vi "Actor Core.vi"(8 "error in":errorcluster, 11 "Controller in":refnum<class "Controller.lvclass">) -> (0 "error out":errorcluster, 3 "Actor out":refnum<class "Actor.lvclass">)   [LabVIEW 2016, in "Controller.lvlib" / "Controller.lvclass"]
doc: "(<B>Filename</B>: Actor Framework.lvlib:Actor.lvclass:Actor Core.vi)\n\nReceives messages to the actor, reacts to them, and initiates any error handling that may shut the actor down.\n\nDescendant classes may override this VI to append parallel tasks for the actor to complete while it handles messages. Overrides use the Call Parent Method node."
uses:
  Controller.lvclass
  C:/Program Files (x86)/National Instruments/LabVIEW 2016/vi.lib/ActorFramework/Actor/Actor.lvclass
  <vilib>/ActorFramework/Actor/Actor.lvclass
  Controls/Controller States.ctl
  Controls/Controller Data.ctl
  <vilib>/ActorFramework/Message Enqueuer/Message Enqueuer.lvclass
  UI/UI/Controls/Start Acquisition.ctl
  <vilib>/userdefined/High Color/IMAQdx.ctl
  Controller.lvclass/Controller.ctl
  Controls/List of Nested Actors.ctl
  UI/UI/UI.lvclass
  <vilib>/ActorFramework/Actor/Actor.lvclass/Actor.ctl
  <vilib>/ActorFramework/Message Enqueuer/Message Enqueuer.lvclass/Message Enqueuer.ctl
  Image Acquisition/Image Acquisition/Image Acquisition.lvclass
  Image Acquisition/Image Acquisition Messages/Start Acq Msg/Start Acq Msg.lvclass/Start Acq Msg.ctl
  Controller Messages/UpdateAcquisitionEnqueuer Msg/UpdateAcquisitionEnqueuer Msg.lvclass/UpdateAcquisitionEnqueuer Msg.ctl
  Tests/Tests/Child Classes/Threshold/Threshold.lvclass
  Tests/Tests/Child Classes/Grayscale/Grayscale.lvclass
  Tests/Tests/Child Classes/Histogram/Histogram.lvclass
  <vilib>/ActorFramework/Report Error Msg/Report Error Msg.lvclass/Report Error Msg.ctl
  <vilib>/ActorFramework/Message Enqueuer/Init from Existing Queue.vi
  <vilib>/ActorFramework/Message Enqueuer/Enqueue.vi
  Image Acquisition/Image Acquisition Messages/Start Acq Msg/Start Acq Msg.lvclass
  C:/Program Files (x86)/National Instruments/LabVIEW 2016/vi.lib/ActorFramework/Message/Message.lvclass
  Controller Messages/UpdateAcquisitionEnqueuer Msg/UpdateAcquisitionEnqueuer Msg.lvclass
  Image Acquisition/Image Acquisition Messages/Stop Acq Msg/Stop Acq Msg.lvclass
  <vilib>/ActorFramework/Report Error Msg/Report Error Msg.lvclass
  <vilib>/ActorFramework/Stop Msg/Stop Msg.lvclass
  <vilib>/ActorFramework/Message Priority Queue/Priority Enqueue.vi
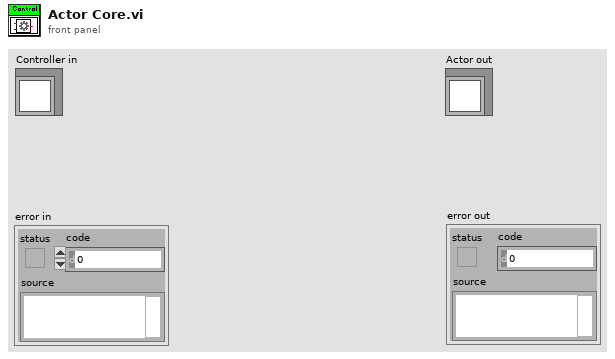
[diagram p1: front panel]
types:
  T1 = typedef "Controller Data.ctl" = cluster{"Controller in":refnum<class "Controller.lvclass">, "Self Enqueuer":refnum<class "Message Enqueuer.lvclass">, "ImgAcq Enqueuer":refnum<class "Message Enqueuer.lvclass">, "UI Enqueuer":refnum<class "Message Enqueuer.lvclass">, "Event Reg Refnum":refnum<event-registration>, "Start Acquisition":T2, "Grayscale Enqueuers":refnum<class "Message Enqueuer.lvclass">[], "HIstogram Enqueuers":refnum<class "Message Enqueuer.lvclass">[], "Threshold Enqueuers":refnum<class "Message Enqueuer.lvclass">[]}
  T2 = typedef "Start Acquisition.ctl" = cluster{"Image Indicator Reference":refnum<vi>, "Start":bool, "Camera":T3}
  T3 = typedef "IMAQdx.ctl" = refnum<k21>
  T4 = typedef "Controller States.ctl" = enum16{"Poll", "Initialize", "Launch-ImgAcqActor", "Stop-ImgAcqActor", "Launch-Threshold", "Launch-Grayscale", "Launch-Histogram", "Stop-Threshold", "Stop-Histogram", "Stop-Grayscale", "Error", "Exit"}
  T5 = typedef "List of Nested Actors.ctl" = enum16{"Threshold", "Grayscale", "Histogram", "UI", "Acquisition"}
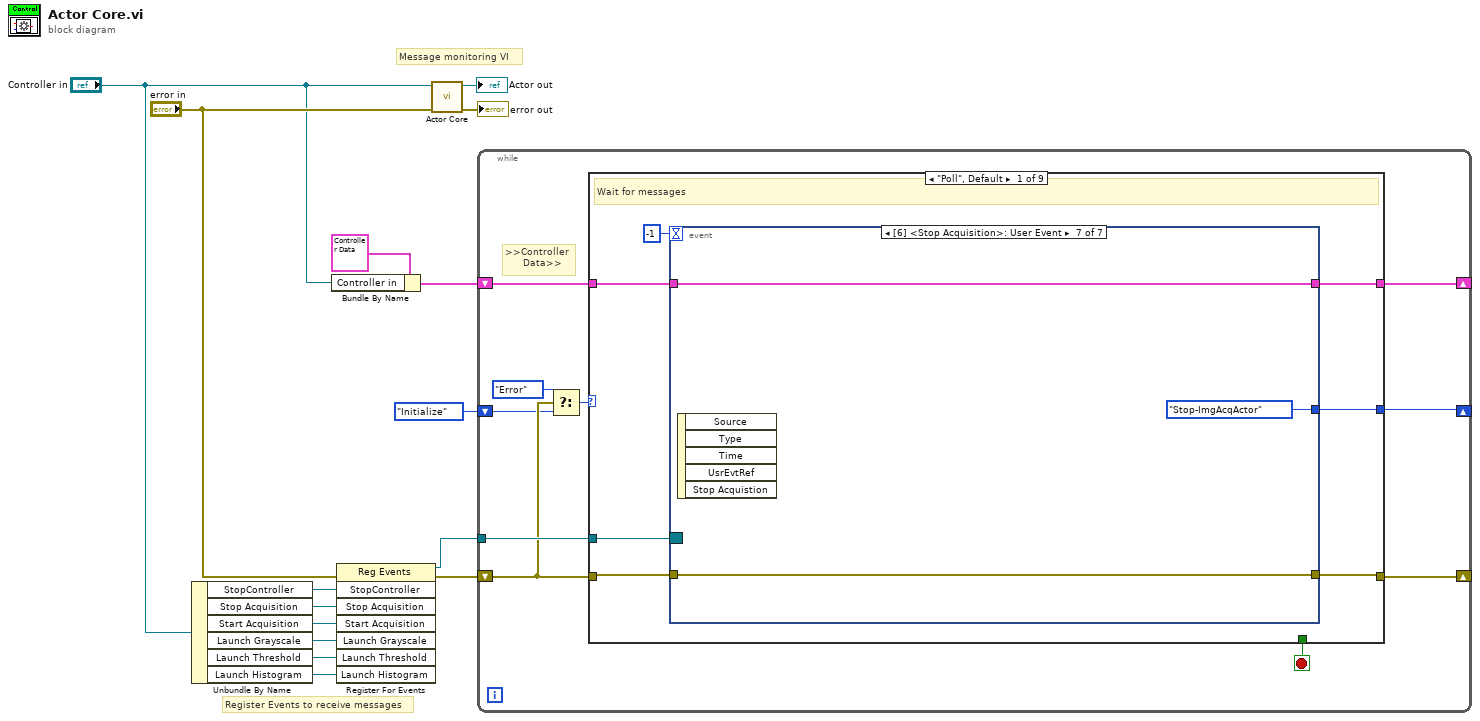
[diagram p0: block diagram]
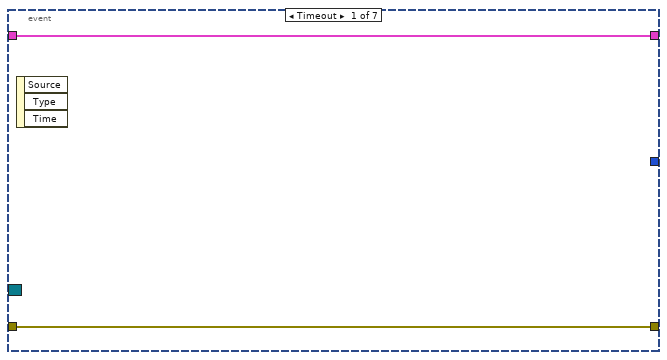
[diagram p2: hidden frame]
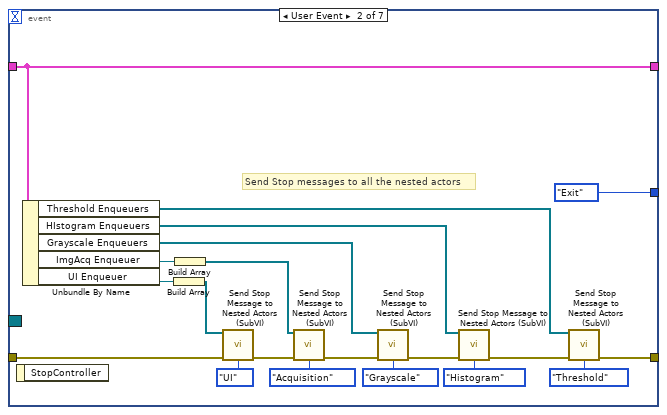
[diagram p3: hidden frame]
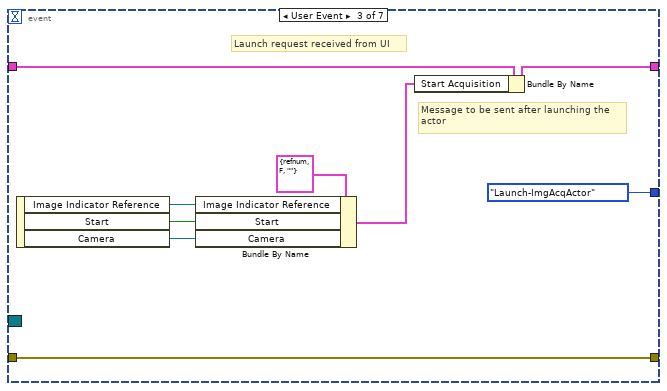
[diagram p4: hidden frame]
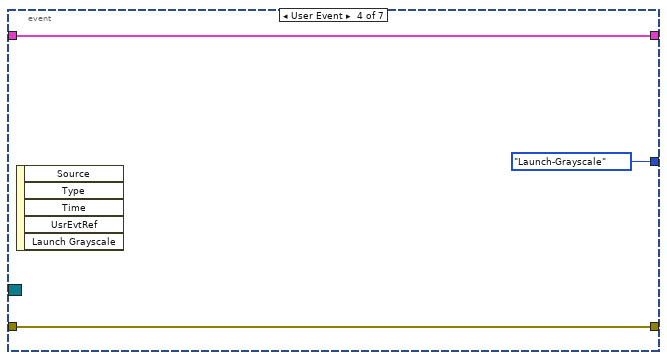
[diagram p5: hidden frame]
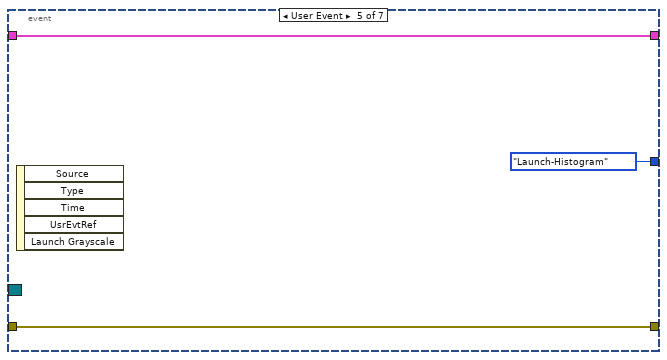
[diagram p6: hidden frame]
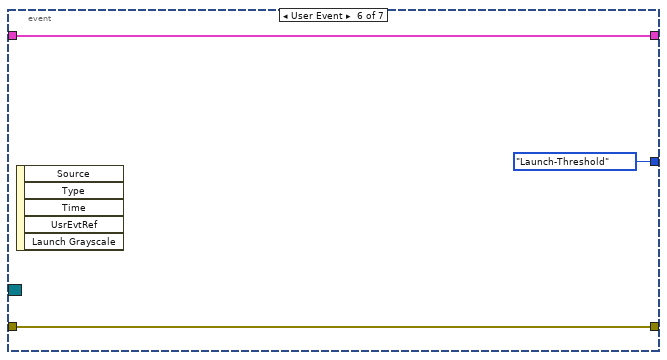
[diagram p7: hidden frame]
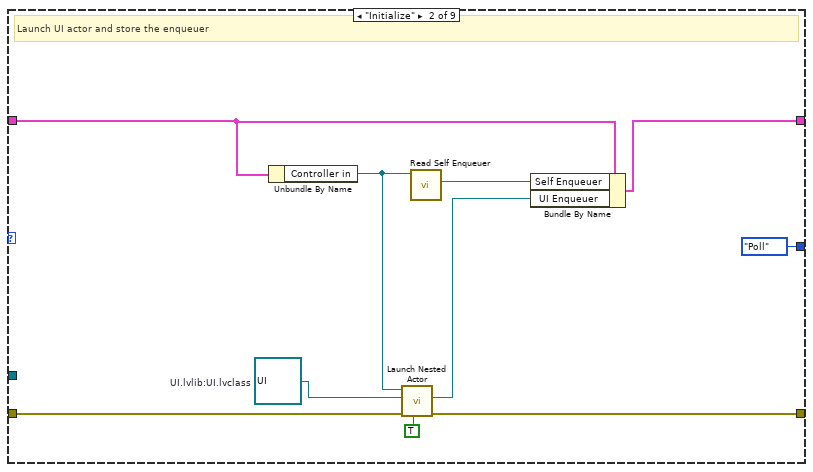
[diagram p8: hidden frame]
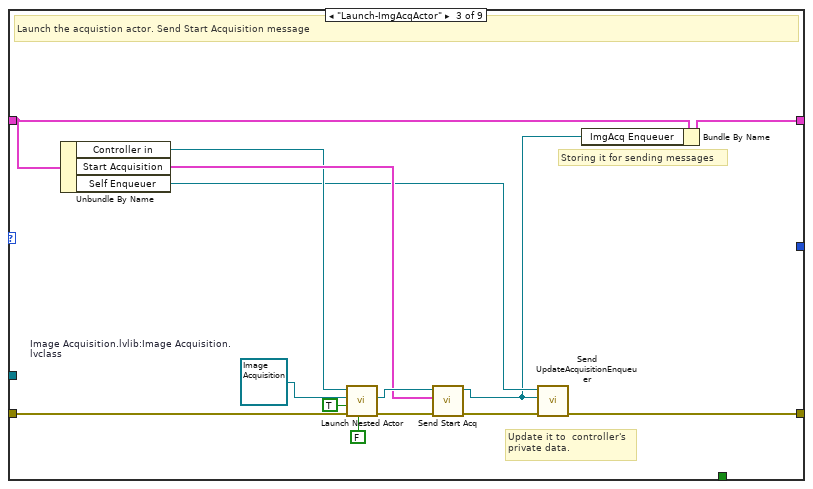
[diagram p9: hidden frame]
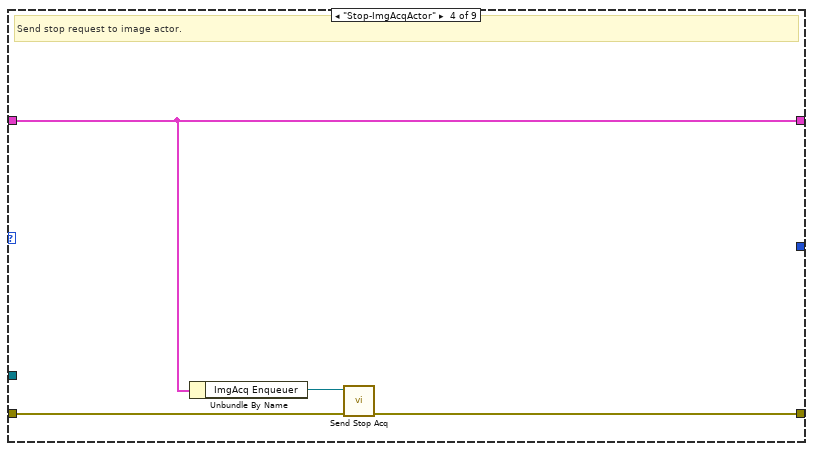
[diagram p10: hidden frame]
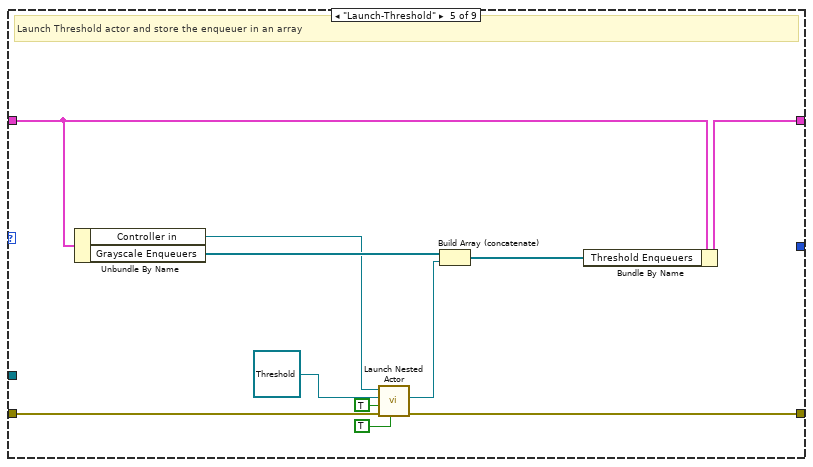
[diagram p11: hidden frame]
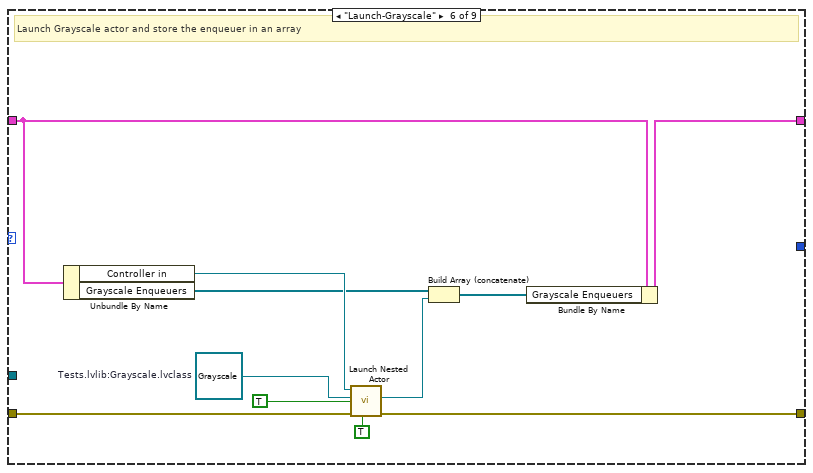
[diagram p12: hidden frame]
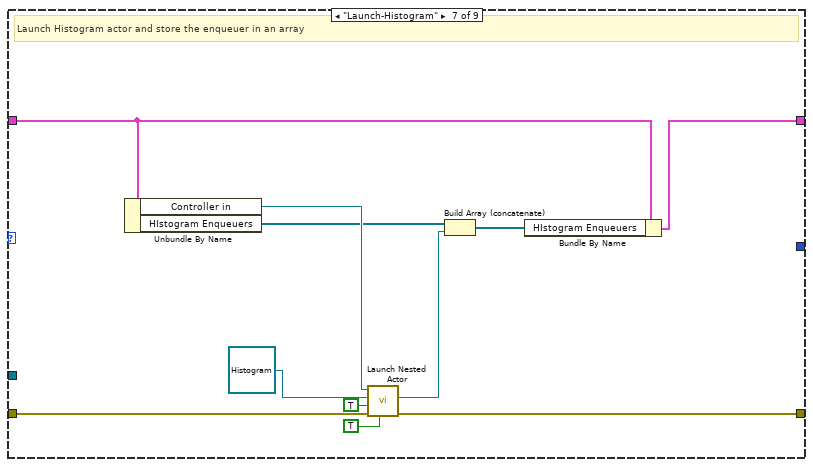
[diagram p13: hidden frame]
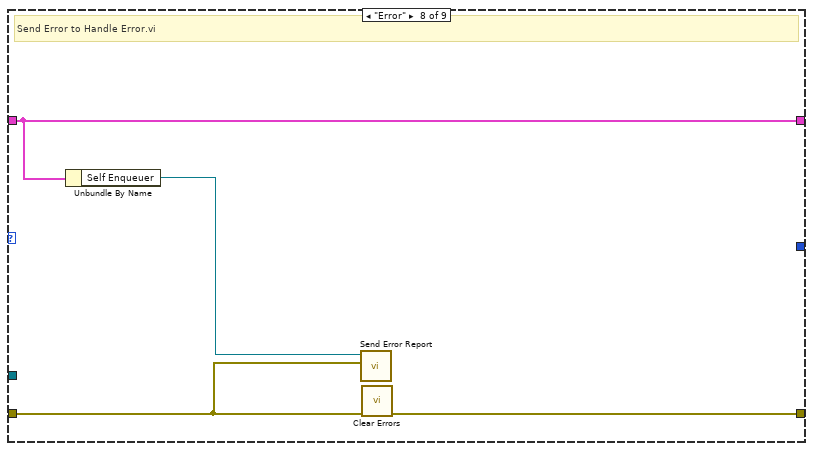
[diagram p14: hidden frame]
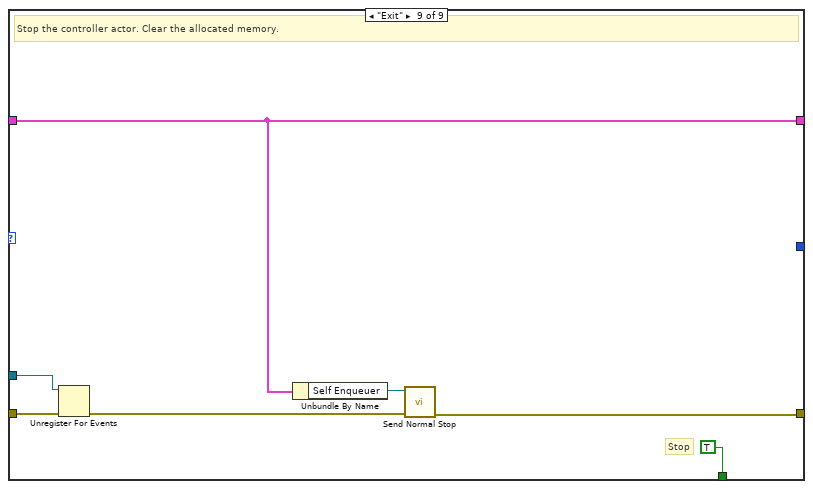
[diagram p15: hidden frame]
diagram:
  # "Message monitoring VI"
  # "Register Events to receive messages"
  n1 = Unbundle By Name("Controller in") -> ("StopController"=w10:refnum<user-event>, "Stop Acquisition"=w9:refnum<user-event>, "Start Acquisition"=w8:refnum<user-event>, "Launch Grayscale"=w4:refnum<user-event>, "Launch Threshold"=w3:refnum<user-event>, "Launch Histogram"=w2:refnum<user-event>)
  n2 = Bundle By Name(cluster=T1 {"Controller in"=refnum, "Self Enqueuer"=refnum, "ImgAcq Enqueuer"=refnum, "UI Enqueuer"=refnum, "Event Reg Refnum"=refnum, "Start Acquisition"={"Image Indicator Reference"=refnum, "Start"=FALSE, "Camera"=""}, "Grayscale Enqueuers"=[], "HIstogram Enqueuers"=[], "Threshold Enqueuers"=[]}, "Controller in"="Controller in") -> (w11:T1)
  n3 = register-events(error in="error in", w10, w9, w8, w4, w3, w2) -> (reference out=w7:refnum<event-registration>, error out=w6:errorcluster)  [unwired: 1 in]
  n4 = call-parent "Actor Core.vi"("error in"="error in", "Actor in"="Controller in") -> ("error out"=→"error out":errorcluster, "Actor out"=→"Actor out":refnum<class "Actor.lvclass">)  [unwired: 8 in]
  n5 = while {
    shift-right: [w24] -> _
    shift-left: Controller_States."Initialize" -> [w18]
    shift-right: [w25] -> _
    shift-left: w6 -> [w19]
    shift-right: [w22] -> _
    shift-left: w11 -> [w23]
    tunnel: w7 -> [w20]
    stop <- w21 stop-if-true
    # ">>Controller\n      Data>>"
    n6 = Select(t=Controller_States."Error", s=w19, f=w18) -> (s? t:f=w17:T4)
    n7 = case shown="\"Poll\", Default" w17 {
      tunnel: w19 -> [w32 w83 w93 w102 w113 w122 w135 w136 w142]
      tunnel: [w31 w82 w90 w101 w112 w121 w134 w139 w144] -> w25
      tunnel: [w30 Controller_States."Poll" _ _ _ _ _ _ _] -> w24
      tunnel: w23 -> [w29 w81 w89 w100 w108 w124 w126 w138 w146]
      tunnel: [w28 w79 w87 w100 w109 w117 w125 w138 w146] -> w22
      tunnel: [_ _ _ _ _ _ _ _ TRUE] -> w21
      tunnel: w20 -> [w27 _ _ _ _ _ _ _ w140]
      frame "Poll", Default {
        # "Wait for messages"
        n8 = event shown="[6] <Stop Acquisition>: User Event" {
          selector: w27 -> [_ _ _ _ _ _ _]
          dyn-events: _ -> [_ _ _ _ _ _ _]
          timeout: -1 -> [_ _ _ _ _ _ _]
          tunnel: w32 -> [w34 w52 w62 w65 w68 w71 w74]
          tunnel: [w34 w38 w62 w65 w68 w71 w74] -> w31
          tunnel: [_ Controller_States."Exit" Controller_States."Launch-ImgAcqActor" Controller_States."Launch-Grayscale" Controller_States."Launch-Histogram" Controller_States."Launch-Threshold" Controller_States."Stop-ImgAcqActor"] -> w30
          tunnel: w29 -> [w33 w51 w61 w64 w67 w70 w73]
          tunnel: [w33 w51 w56 w64 w67 w70 w73] -> w28
          event Timeout {
            n9 = event-data() -> ()  [unwired: 1 in, 3 out]
          }
          event User Event {
            # "Send Stop messages to all the nested actors"
            n10 = event-data() -> ()  [unwired: 1 in, 1 out]
            n11 = Unbundle By Name(w51) -> ("Threshold Enqueuers"=w41:refnum<class "Message Enqueuer.lvclass">[], "HIstogram Enqueuers"=w42:refnum<class "Message Enqueuer.lvclass">[], "Grayscale Enqueuers"=w43:refnum<class "Message Enqueuer.lvclass">[], "ImgAcq Enqueuer"=w46:refnum<class "Message Enqueuer.lvclass">, "UI Enqueuer"=w50:refnum<class "Message Enqueuer.lvclass">)
            n12 = Build Array(w50) -> (w49:refnum<class "Message Enqueuer.lvclass">[])
            n13 = Build Array(w46) -> (w45:refnum<class "Message Enqueuer.lvclass">[])
            n14 = call "Send Stop Message to Nested Actors (SubVI).vi"("Grayscale Enqueuers"=w49, "error in (no error)"=w52, "Target Actor Enqueuers"=List_of_Nested_Actors."UI") -> ("error out"=w44:errorcluster)  [unwired: 12 in]
            n15 = call "Send Stop Message to Nested Actors (SubVI).vi"("Grayscale Enqueuers"=w45, "error in (no error)"=w44, "Target Actor Enqueuers"=List_of_Nested_Actors."Acquisition") -> ()  [unwired: 12 in, 1 out]
            n16 = call "Send Stop Message to Nested Actors (SubVI).vi"("Grayscale Enqueuers"=w43, "error in (no error)"=w44, "Target Actor Enqueuers"=List_of_Nested_Actors."Grayscale") -> ("error out"=w39:errorcluster)  [unwired: 12 in]
            n17 = call "Send Stop Message to Nested Actors (SubVI).vi"("Grayscale Enqueuers"=w42, "error in (no error)"=w39, "Target Actor Enqueuers"=List_of_Nested_Actors."Histogram") -> ("error out"=w40:errorcluster)  [unwired: 12 in]
            n18 = call "Send Stop Message to Nested Actors (SubVI).vi"("Grayscale Enqueuers"=w41, "error in (no error)"=w40, "Target Actor Enqueuers"=List_of_Nested_Actors."Threshold") -> ("error out"=w38:errorcluster)  [unwired: 12 in]
          }
          event User Event {
            # "Launch request received from UI"
            # "Message to be sent after launching the\nactor"
            n19 = event-data() -> ("Image Indicator Reference"=w57:refnum<vi>, "Start"=w58:bool, "Camera"=w54:T3)  [unwired: 1 in]
            n20 = Bundle By Name(cluster=T2 {"Image Indicator Reference"=refnum, "Start"=FALSE, "Camera"=""} ("Start Acquisition"), "Image Indicator Reference"=w57, "Start"=w58, "Camera"=w54) -> (w55:T2)
            n21 = Bundle By Name(cluster=w61, "Start Acquisition"=w55) -> (w56:T1)
          }
          event User Event {
            n22 = event-data() -> ()  [unwired: 1 in, 5 out]
          }
          event User Event {
            n23 = event-data() -> ()  [unwired: 1 in, 5 out]
          }
          event User Event {
            n24 = event-data() -> ()  [unwired: 1 in, 5 out]
          }
          event User Event {
            n25 = event-data() -> ()  [unwired: 1 in, 5 out]
          }
        }
      }
      frame "Initialize" {
        w78 = refnum<class "UI.lvclass"> refnum  # UI.lvlib:UI.lvclass
        # "Launch UI actor and store the enqueuer"
        n26 = Unbundle By Name(w81) -> ("Controller in"=w77:refnum<class "Controller.lvclass">)
        n27 = call <vilib>:"Launch Nested Actor.vi"("Open Actor Core front panel? (F)"=TRUE, "error in (no error)"=w83, "Nested Actor"=w78, "Caller Actor in"=w77) -> ("error out"=w82:errorcluster, "Nested Actor's Enqueuer"=w75:refnum<class "Message Enqueuer.lvclass">)  [unwired: 5 in, 1 out]
        n28 = call <vilib>:"Read Self Enqueuer.vi"("Actor"=w77) -> ("Self Enqueuer"=w80:refnum<class "Message Enqueuer.lvclass">)  [unwired: 10 in]
        n29 = Bundle By Name(cluster=w81, "Self Enqueuer"=w80, "UI Enqueuer"=w75) -> (w79:T1)
      }
      frame "Launch-ImgAcqActor" {
        w92 = refnum<class "Image Acquisition.lvclass"> refnum  # Image Acquisition.lvlib:Image Acquisition.lvclass
        # "Storing it for sending messages"
        # "Update it to  controller's\nprivate data."
        # "Launch the acquistion actor. Send Start Acquisition message"
        n30 = Unbundle By Name(w89) -> ("Controller in"=w94:refnum<class "Controller.lvclass">, "Start Acquisition"=w96:T2, "Self Enqueuer"=w88:refnum<class "Message Enqueuer.lvclass">)
        n31 = call <vilib>:"Launch Nested Actor.vi"("Open Actor Core front panel? (F)"=FALSE, "error in (no error)"=w93, "Auto-stop? (T)"=TRUE, "Nested Actor"=w92, "Caller Actor in"=w94) -> ("error out"=w98:errorcluster, "Nested Actor's Enqueuer"=w97:refnum<class "Message Enqueuer.lvclass">)  [unwired: 4 in, 1 out]
        n32 = call "Send Start Acq.vi"("error in (no error)"=w98, "Acquistion Parameters"=w96, "Message Enqueuer"=w97) -> ("error out"=w91:errorcluster, "Message Enqueuer out"=w86:refnum<class "Message Enqueuer.lvclass">)  [unwired: 7 in]
        n33 = call "Send UpdateAcquisitionEnqueuer.vi"("error in (no error)"=w91, "Acquisition Enqueuer"=w86, "Message Enqueuer"=w88) -> ("error out"=w90:errorcluster)  [unwired: 7 in, 1 out]
        n34 = Bundle By Name(cluster=w89, "ImgAcq Enqueuer"=w86) -> (w87:T1)
      }
      frame "Stop-ImgAcqActor" {
        # "Send stop request to image actor."
        n35 = Unbundle By Name(w100) -> ("ImgAcq Enqueuer"=w99:refnum<class "Message Enqueuer.lvclass">)
        n36 = call "Send Stop Acq.vi"("error in (no error)"=w102, "Message Enqueuer"=w99) -> ("error out"=w101:errorcluster)  [unwired: 8 in, 1 out]
      }
      frame "Launch-Threshold" {
        # "Launch Threshold actor and store the enqueuer in an array"
        n37 = Unbundle By Name(w108) -> ("Controller in"=w106:refnum<class "Controller.lvclass">, "Grayscale Enqueuers"=w111:refnum<class "Message Enqueuer.lvclass">[])
        n38 = call <vilib>:"Launch Nested Actor.vi"("Open Actor Core front panel? (F)"=TRUE, "error in (no error)"=w113, "Auto-stop? (T)"=TRUE, "Nested Actor"=refnum<class "Threshold.lvclass"> refnum ("Tests.lvlib:Threshold.lvclass"), "Caller Actor in"=w106) -> ("error out"=w112:errorcluster, "Nested Actor's Enqueuer"=w107:refnum<class "Message Enqueuer.lvclass">)  [unwired: 4 in, 1 out]
        n39 = Build Array (concatenate)(w111, w107) -> (w110:refnum<class "Message Enqueuer.lvclass">[])
        n40 = Bundle By Name(cluster=w108, "Threshold Enqueuers"=w110) -> (w109:T1)
      }
      frame "Launch-Grayscale" {
        w118 = refnum<class "Grayscale.lvclass"> refnum  # Tests.lvlib:Grayscale.lvclass
        # "Launch Grayscale actor and store the enqueuer in an array"
        n41 = Unbundle By Name(w124) -> ("Controller in"=w123:refnum<class "Controller.lvclass">, "Grayscale Enqueuers"=w116:refnum<class "Message Enqueuer.lvclass">[])
        n42 = call <vilib>:"Launch Nested Actor.vi"("Open Actor Core front panel? (F)"=TRUE, "error in (no error)"=w122, "Auto-stop? (T)"=TRUE, "Nested Actor"=w118, "Caller Actor in"=w123) -> ("error out"=w121:errorcluster, "Nested Actor's Enqueuer"=w115:refnum<class "Message Enqueuer.lvclass">)  [unwired: 4 in, 1 out]
        n43 = Build Array (concatenate)(w116, w115) -> (w114:refnum<class "Message Enqueuer.lvclass">[])
        n44 = Bundle By Name(cluster=w124, "Grayscale Enqueuers"=w114) -> (w117:T1)
      }
      frame "Launch-Histogram" {
        # "Launch Histogram actor and store the enqueuer in an array"
        n45 = Unbundle By Name(w126) -> ("Controller in"=w133:refnum<class "Controller.lvclass">, "HIstogram Enqueuers"=w129:refnum<class "Message Enqueuer.lvclass">[])
        n46 = call <vilib>:"Launch Nested Actor.vi"("Open Actor Core front panel? (F)"=TRUE, "error in (no error)"=w135, "Auto-stop? (T)"=TRUE, "Nested Actor"=refnum<class "Histogram.lvclass"> refnum ("Tests.lvlib:Histogram.lvclass"), "Caller Actor in"=w133) -> ("error out"=w134:errorcluster, "Nested Actor's Enqueuer"=w128:refnum<class "Message Enqueuer.lvclass">)  [unwired: 4 in, 1 out]
        n47 = Build Array (concatenate)(w129, w128) -> (w127:refnum<class "Message Enqueuer.lvclass">[])
        n48 = Bundle By Name(cluster=w126, "HIstogram Enqueuers"=w127) -> (w125:T1)
      }
      frame "Error" {
        # "Send Error to Handle Error.vi"
        n49 = Unbundle By Name(w138) -> ("Self Enqueuer"=w137:refnum<class "Message Enqueuer.lvclass">)
        n50 = call <vilib>:"Send Error Report.vi"("Error From Sender"=w136, "Message Enqueuer"=w137) -> ()  [unwired: 9 in, 1 out]
        n51 = call <vilib>:"Clear Errors.vi"("error in (no error)"=w136) -> ("error out"=w139:errorcluster)  [unwired: 5 in, 1 out]
      }
      frame "Exit" {
        # "Stop"
        # "Stop the controller actor. Clear the allocated memory."
        n52 = Unregister For Events(event registration refnum=w140, error in=w142) -> (error out=w141:errorcluster)
        n53 = Unbundle By Name(w146) -> ("Self Enqueuer"=w145:refnum<class "Message Enqueuer.lvclass">)
        n54 = call <vilib>:"Send Normal Stop.vi"("error in (no error)"=w141, "Message Enqueuer"=w145) -> ("error out"=w144:errorcluster)  [unwired: 9 in]
      }
    }
  }
